vi "Robot Main.vi"() -> ()   [LabVIEW 2013]
uses:
  <vilib>/Rock Robotics/WPI/DriverStation/WPI_DriverStationRobotMode2.ctl
  Robot/Logical Systems/Drive Train/Drive Train Class/Drive Train Status.ctl
  Robot/Robot Actors/System Actor/System Actor Class/System Status.ctl
  Robot/Robot Actors/Command/Command Class/Command Status.ctl
  Robot/Robot Actors/Command/Command Class/Command States.ctl
  Robot/Logical Systems/Driver/Driver-Logical/Driver Status.ctl
  Robot/Logical Systems/XBox Controller/Xbox Controller.ctl
  Robot/Virtual Systems/XBox Controller/XBox Controller Class/Joystick.ctl
  Robot/Logical Systems/Drive Train/Drive Train Messages/Write Drive Train Status Ref Msg/Write Drive Train Status Ref Msg.lvclass/Write Drive Train Status Ref Msg.ctl
  <vilib>/ActorFramework/Message Enqueuer/Message Enqueuer.lvclass/Message Enqueuer.ctl
  Robot/Robot Actors/System Actor/System Actor Messages/Write System Status Ref Msg/Write System Status Ref Msg.lvclass/Write System Status Ref Msg.ctl
  Robot/Logical Systems/Driver/Driver Messages/Write Driver Status Ref Msg/Write Driver Status Ref Msg.lvclass/Write Driver Status Ref Msg.ctl
  <vilib>/ActorFramework/Message Enqueuer/Enqueue.vi
  Robot Global.vi
  <vilib>/ActorFramework/Message Priority Queue/Priority Enqueue.vi
  Robot/Logical Systems/Drive Train/Drive Train Messages/Write Drive Train Status Ref Msg/Write Drive Train Status Ref Msg.lvclass
  Robot/Robot Actors/System Actor/System Actor Messages/Write System Status Ref Msg/Write System Status Ref Msg.lvclass
  Robot/Logical Systems/Driver/Driver Messages/Write Driver Status Ref Msg/Write Driver Status Ref Msg.lvclass
  Robot/Logical Systems/Drive Train/Drive Train Class/Drive Train.lvclass
  Robot/Robot Actors/Command/Command Class/Command.lvclass
  Robot/Robot Actors/System Actor/System Actor Class/System Actor.lvclass
  Robot/Logical Systems/XBox Controller/XBox Controller Class/Xbox Controller.lvlib
  Robot/Logical Systems/Driver/Driver-Logical/Driver.lvclass
panel:
  in  "Run Tele?":bool
  in  "milliseconds to wait":u32=1000 step=50
  in  "Systems":enum32{"Drive Train", "Driver"}(tab)
  in  "Drive Train - System Status":T1
  in  "Drive Train Status":T4 {"Right Power Setpoint" min=-1.0 max=1.0 step=0.1 scale=-1.0..1.0; "Left Power Setpoint" min=-1.0 max=1.0 step=0.1 scale=-1.0..1.0; "Right Power" min=-1.0 max=1.0 step=0.1 scale=-1.0..1.0; "Left Power" min=-1.0 max=1.0 step=0.1 scale=-1.0..1.0}
  in  "Driver - System Status":T1
  in  "Driver Status":T5 {"Current Xbox Controller"."Right Joystick"."Right" min=-1.0 max=1.0 step=0.1 scale=-1.0..1.0; "Current Xbox Controller"."Right Joystick"."Forward" min=-1.0 max=1.0 step=0.1 scale=-1.0..1.0; "Current Xbox Controller"."Left Joystick"."Right" min=-1.0 max=1.0 step=0.1 scale=-1.0..1.0; "Current Xbox Controller"."Left Joystick"."Forward" min=-1.0 max=1.0 step=0.1 scale=-1.0..1.0}
  in  "Finish Button":bool
  in  "Robot Mode":T8=enum."Teleop Enabled"
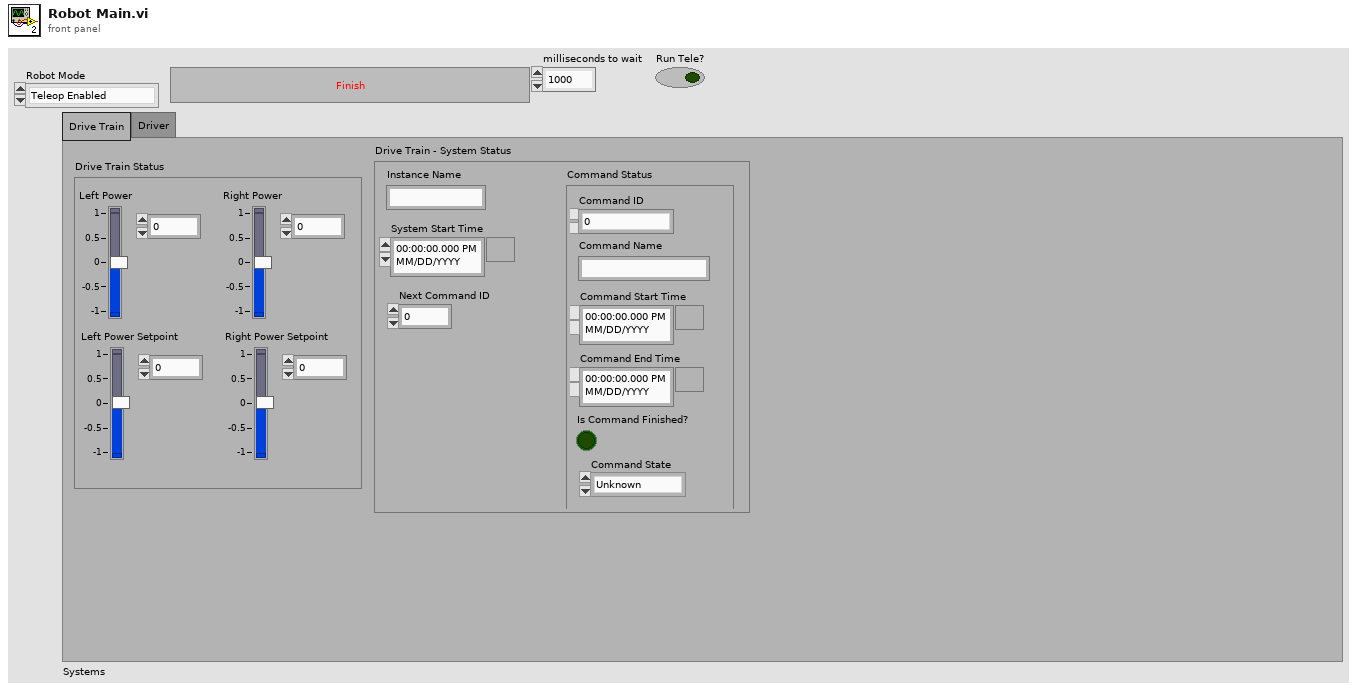
[diagram p1: front panel]
types:
  T1 = typedef "Robot Actors.lvlib/System Actor.lvlib/System Actor.lvclass/System Status.ctl" = cluster{"Instance Name":string, "Command Status":T2, "System Start Time":timestamp, "Next Command ID":dbl}
  T2 = typedef "Robot Actors.lvlib/Command.lvlib/Command.lvclass/Command Status.ctl" = cluster{"Command Name":string, "Command Start Time":timestamp, "Command End Time":timestamp, "Is Command Finished?":bool, "Command ID":dbl, "Command State":T3}
  T3 = typedef "Robot Actors.lvlib/Command.lvlib/Command.lvclass/Command States.ctl" = enum16{"Unknown", "Started", "Stopped", "Finished"}
  T4 = typedef "Logical Systems.lvlib/Drive Train.lvlib/Drive Train.lvclass/Drive Train Status.ctl" = cluster{"Left Power":dbl, "Right Power":dbl, "Left Power Setpoint":dbl, "Right Power Setpoint":dbl}
  T5 = typedef "Logical Systems.lvlib/Driver.lvlib/Driver.lvclass/Driver Status.ctl" = cluster{"Current Xbox Controller":T6}
  T6 = typedef "Logical Systems.lvlib/Xbox Controller.lvlib/Xbox Controller.ctl" = cluster{"Left Joystick":T7, "Right Joystick":T7}
  T7 = typedef "Logical Systems.lvlib/Xbox Controller.lvlib/Joystick.ctl" = cluster{"Forward":dbl, "Right":dbl}
  T8 = typedef "WPI_DriverStationRobotMode2.ctl" = enum16{"Autonomous Disabled", "Autonomous Enabled", "Teleop Disabled", "Teleop Enabled", "Timeout", "Finish", "Test Disabled", "Test Enabled"}
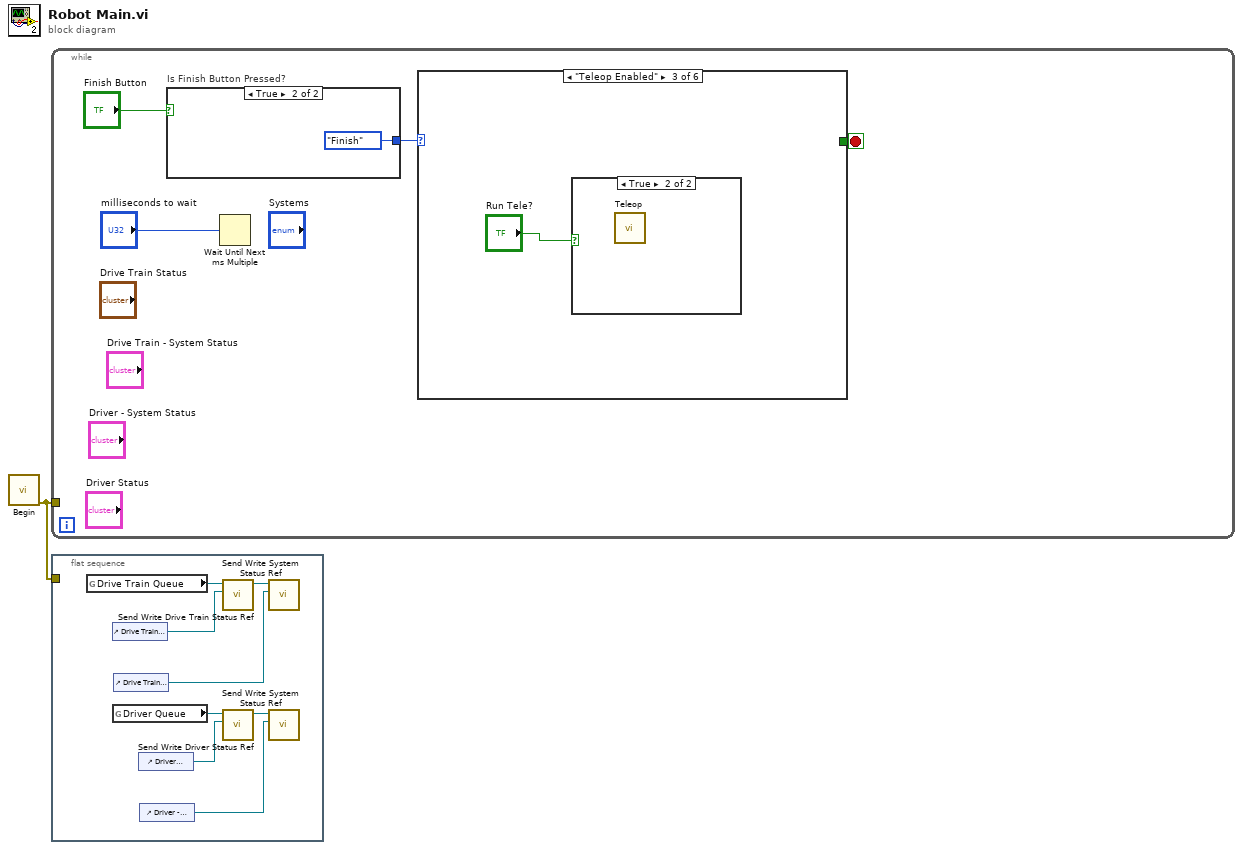
[diagram p0: block diagram]
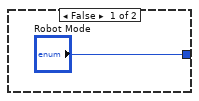
[diagram p2: hidden frame]
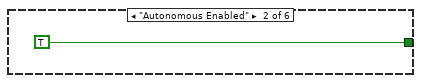
[diagram p4: hidden frame]
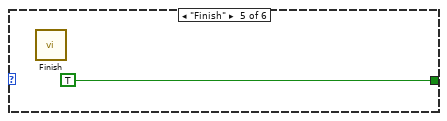
[diagram p7: hidden frame]
diagram:
  n1 = call "Begin.vi"() -> ("error out"=w1:errorcluster)  [unwired: 11 in]
  n2 = while {
    tunnel: w1 -> [_]
    stop <- w4 stop-if-true
    n3 = case "Is Finish Button Pressed?" shown="True" "Finish Button" {
      tunnel: ["Robot Mode" WPI_DriverStationRobotMode2."Finish" ("Robot Mode")] -> w5
      frame False {
      }
      frame True {
      }
    }
    n4 = Wait Until Next ms Multiple(millisecond multiple="milliseconds to wait") -> ()  [unwired: 1 out]
    n5 = case shown="\"Teleop Enabled\"" w5 {
      tunnel: [_ TRUE _ _ TRUE _] -> w4
      frame "Autonomous Disabled", "Teleop Disabled" {
      }
      frame "Autonomous Enabled" {
      }
      frame "Teleop Enabled" {
        n6 = case shown="True" "Run Tele?" {
          frame False {
          }
          frame True {
            n7 = call "Teleop.vi"() -> ()  [unwired: 12 in]
          }
        }
      }
      frame "Timeout" {
      }
      frame "Finish" {
        n8 = call "Finish.vi"() -> ()  [unwired: 12 in]
      }
      frame "Test Disabled", "Test Enabled" {
      }
    }
  }
  n9 = flat-sequence {
    tunnel: w1 -> [_]
    frame #0 {
      n10 = global read "Robot Global.vi" "Drive Train Queue"() -> (w18:refnum<class "Message Enqueuer.lvclass">)
      n11 = control-ref of="Drive Train Status"() -> (w17:refnum<vi>)
      n12 = global read "Robot Global.vi" "Driver Queue"() -> (w14:refnum<class "Message Enqueuer.lvclass">)
      n13 = control-ref of="Drive Train - System Status"() -> (w15:refnum<vi>)
      n14 = control-ref of="Driver Status"() -> (w13:refnum<vi>)
      n15 = control-ref of="Driver - System Status"() -> (w11:refnum<vi>)
      n16 = call "Send Write Drive Train Status Ref.vi"("Drive Train Status Ref"=w17, "Message Enqueuer"=w18) -> ("Message Enqueuer out"=w16:refnum<class "Message Enqueuer.lvclass">)  [unwired: 8 in, 1 out]
      n17 = call "Send Write Driver Status Ref.vi"("Driver Status Ref"=w13, "Message Enqueuer"=w14) -> ("Message Enqueuer out"=w12:refnum<class "Message Enqueuer.lvclass">)  [unwired: 8 in, 1 out]
      n18 = call "Send Write System Status Ref.vi"("System Status Ref"=w15, "Message Enqueuer"=w16) -> ()  [unwired: 8 in, 2 out]
      n19 = call "Send Write System Status Ref.vi"("System Status Ref"=w11, "Message Enqueuer"=w12) -> ()  [unwired: 8 in, 2 out]
    }
  }
